vi "Machine Opt.vi"(8 "error in (no error)":errorcluster caption="错误输入（无错误）", 11 "Machine Opt":T1=enum."送电启动") -> (0 "error out":errorcluster caption="错误输出", 3 "Output(U8)":u8)   [LabVIEW 2012]
uses:
  Machine Opt.ctl
  Relay Name.ctl
  OffOn.ctl
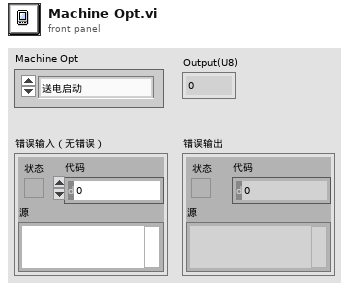
[diagram p1: front panel]
types:
  T1 = typedef "Machine Opt.ctl" = enum16{"初始化", "送电启动", "送电关闭", "液压站启动", "液压站停止", "润滑启动", "润滑停止", "冷却启动", "冷却停止", "快进启动", "快进停止", "工进启动", "工进停止", "快退启动", "快退停止", "报警启动", "报警停止"}
  T2 = typedef "OffOn.ctl" = enum16{"Off", "On"}
  T3 = typedef "Relay Name.ctl" = enum8{"送电", "液压站", "润滑电机", "冷却电机", "滑台快进", "滑台工进", "滑台快退", "报警指示灯"}
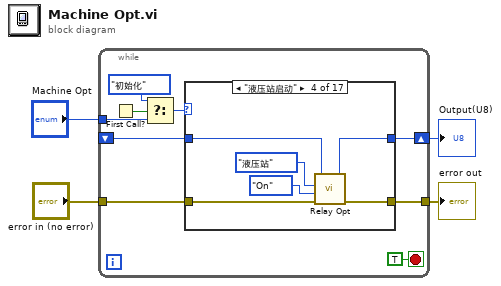
[diagram p0: block diagram]
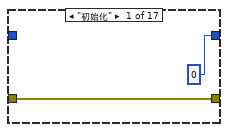
[diagram p2: hidden frame]
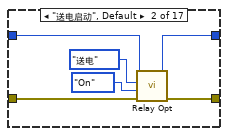
[diagram p3: hidden frame]
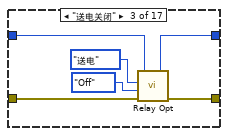
[diagram p4: hidden frame]
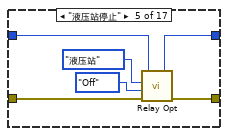
[diagram p5: hidden frame]
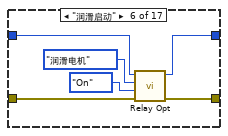
[diagram p6: hidden frame]
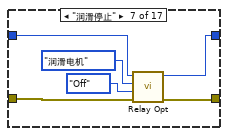
[diagram p7: hidden frame]
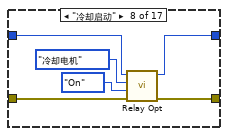
[diagram p8: hidden frame]
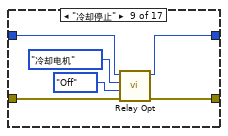
[diagram p9: hidden frame]
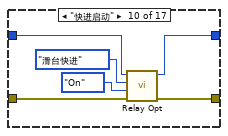
[diagram p10: hidden frame]
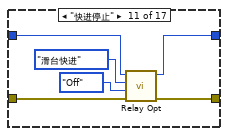
[diagram p11: hidden frame]
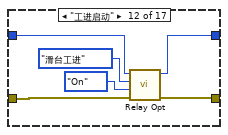
[diagram p12: hidden frame]
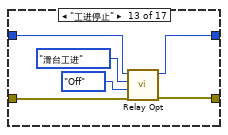
[diagram p13: hidden frame]
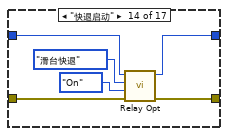
[diagram p14: hidden frame]
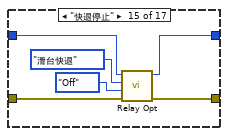
[diagram p15: hidden frame]
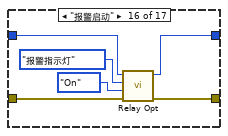
[diagram p16: hidden frame]
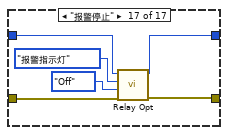
[diagram p17: hidden frame]
diagram:
  n1 = while {
    tunnel: "error in (no error)" -> [w13]
    tunnel: [w12] -> w3
    tunnel: "Machine Opt" -> [w6]
    shift-right: [w10] -> w1
    shift-left: _ -> [w9]
    stop <- TRUE stop-if-true
    n2 = First Call?() -> (First Call?: T/F=w8:bool)
    n3 = Select(t=Machine_Opt."初始化" ("Machine Opt"), s=w8, f=w6) -> (s? t:f=w5:T1)
    n4 = case shown="\"液压站启动\"" w5 {
      tunnel: w13 -> [w14 w19 w27 w31 w37 w43 w49 w55 w60 w67 w73 w79 w84 w91 w96 w103 w106]
      tunnel: [w14 w18 w26 w30 w36 w42 w48 w54 w61 w66 w72 w78 w85 w90 w97 w102 w107] -> w12
      tunnel: [u8 0 ("Output(U8)") w17 w25 w28 w34 w40 w47 w53 w59 w65 w71 w77 w82 w89 w95 w101 w108] -> w10
      tunnel: w9 -> [_ w16 w24 w29 w35 w41 w46 w52 w58 w64 w70 w76 w83 w88 w94 w100 w109]
      frame "初始化" {
      }
      frame "送电启动", Default {
        n5 = call "Relay Opt.vi"("error in (no error)"=w19, "OnOff"=OffOn."On", "Relay"=Relay_Name."送电", "Input(U8)"=w16) -> ("error out"=w18:errorcluster, "Output(U8)"=w17:u8)  [unwired: 6 in]
      }
      frame "送电关闭" {
        n6 = call "Relay Opt.vi"("error in (no error)"=w27, "OnOff"=OffOn."Off", "Relay"=Relay_Name."送电", "Input(U8)"=w24) -> ("error out"=w26:errorcluster, "Output(U8)"=w25:u8)  [unwired: 6 in]
      }
      frame "液压站启动" {
        n7 = call "Relay Opt.vi"("error in (no error)"=w31, "OnOff"=OffOn."On", "Relay"=Relay_Name."液压站", "Input(U8)"=w29) -> ("error out"=w30:errorcluster, "Output(U8)"=w28:u8)  [unwired: 6 in]
      }
      frame "液压站停止" {
        n8 = call "Relay Opt.vi"("error in (no error)"=w37, "OnOff"=OffOn."Off", "Relay"=Relay_Name."液压站", "Input(U8)"=w35) -> ("error out"=w36:errorcluster, "Output(U8)"=w34:u8)  [unwired: 6 in]
      }
      frame "润滑启动" {
        n9 = call "Relay Opt.vi"("error in (no error)"=w43, "OnOff"=OffOn."On", "Relay"=Relay_Name."润滑电机", "Input(U8)"=w41) -> ("error out"=w42:errorcluster, "Output(U8)"=w40:u8)  [unwired: 6 in]
      }
      frame "润滑停止" {
        n10 = call "Relay Opt.vi"("error in (no error)"=w49, "OnOff"=OffOn."Off", "Relay"=Relay_Name."润滑电机", "Input(U8)"=w46) -> ("error out"=w48:errorcluster, "Output(U8)"=w47:u8)  [unwired: 6 in]
      }
      frame "冷却启动" {
        n11 = call "Relay Opt.vi"("error in (no error)"=w55, "OnOff"=OffOn."On", "Relay"=Relay_Name."冷却电机", "Input(U8)"=w52) -> ("error out"=w54:errorcluster, "Output(U8)"=w53:u8)  [unwired: 6 in]
      }
      frame "冷却停止" {
        n12 = call "Relay Opt.vi"("error in (no error)"=w60, "OnOff"=OffOn."Off", "Relay"=Relay_Name."冷却电机", "Input(U8)"=w58) -> ("error out"=w61:errorcluster, "Output(U8)"=w59:u8)  [unwired: 6 in]
      }
      frame "快进启动" {
        n13 = call "Relay Opt.vi"("error in (no error)"=w67, "OnOff"=OffOn."On", "Relay"=Relay_Name."滑台快进", "Input(U8)"=w64) -> ("error out"=w66:errorcluster, "Output(U8)"=w65:u8)  [unwired: 6 in]
      }
      frame "快进停止" {
        n14 = call "Relay Opt.vi"("error in (no error)"=w73, "OnOff"=OffOn."Off", "Relay"=Relay_Name."滑台快进", "Input(U8)"=w70) -> ("error out"=w72:errorcluster, "Output(U8)"=w71:u8)  [unwired: 6 in]
      }
      frame "工进启动" {
        n15 = call "Relay Opt.vi"("error in (no error)"=w79, "OnOff"=OffOn."On", "Relay"=Relay_Name."滑台工进", "Input(U8)"=w76) -> ("error out"=w78:errorcluster, "Output(U8)"=w77:u8)  [unwired: 6 in]
      }
      frame "工进停止" {
        n16 = call "Relay Opt.vi"("error in (no error)"=w84, "OnOff"=OffOn."Off", "Relay"=Relay_Name."滑台工进", "Input(U8)"=w83) -> ("error out"=w85:errorcluster, "Output(U8)"=w82:u8)  [unwired: 6 in]
      }
      frame "快退启动" {
        n17 = call "Relay Opt.vi"("error in (no error)"=w91, "OnOff"=OffOn."On", "Relay"=Relay_Name."滑台快退", "Input(U8)"=w88) -> ("error out"=w90:errorcluster, "Output(U8)"=w89:u8)  [unwired: 6 in]
      }
      frame "快退停止" {
        n18 = call "Relay Opt.vi"("error in (no error)"=w96, "OnOff"=OffOn."Off", "Relay"=Relay_Name."滑台快退", "Input(U8)"=w94) -> ("error out"=w97:errorcluster, "Output(U8)"=w95:u8)  [unwired: 6 in]
      }
      frame "报警启动" {
        n19 = call "Relay Opt.vi"("error in (no error)"=w103, "OnOff"=OffOn."On", "Relay"=Relay_Name."报警指示灯", "Input(U8)"=w100) -> ("error out"=w102:errorcluster, "Output(U8)"=w101:u8)  [unwired: 6 in]
      }
      frame "报警停止" {
        n20 = call "Relay Opt.vi"("error in (no error)"=w106, "OnOff"=OffOn."Off", "Relay"=Relay_Name."报警指示灯", "Input(U8)"=w109) -> ("error out"=w107:errorcluster, "Output(U8)"=w108:u8)  [unwired: 6 in]
      }
    }
  }
  "error out" <- w3
  "Output(U8)" <- w1
